vi "Write Subdiagram Labels.vi"(8 "Error In":errorcluster, 11 "DisableStructure In":refnum<vi>) -> (0 "Error Out":errorcluster, 3 "DisableStructure Out":refnum<vi>)   [LabVIEW 2017, in "Toolkit.lvlib"]
uses:
  Toolkit.lvlib
  Typedefs/Grave Frames.ctl
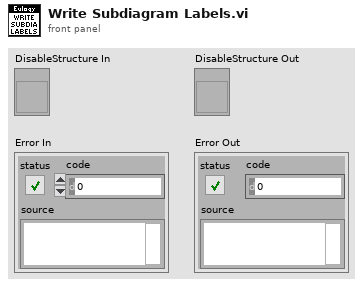
[diagram p1: front panel]
types:
  T1 = typedef "Toolkit.lvlib/Grave Frames.ctl" = enum16{"Corpse", "Spirit"}
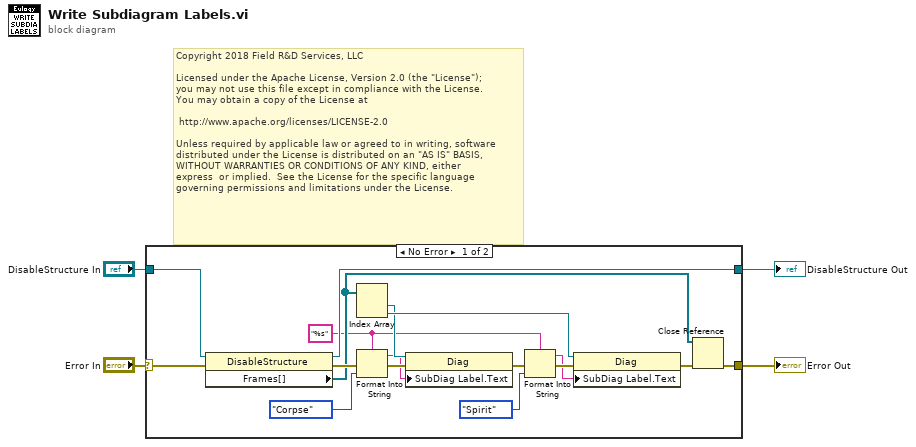
[diagram p0: block diagram]
diagram:
  # "Copyright 2018 Field R&D Services, LLC\n\nLicensed under the Apache License, Version 2.0 (the \"License\");\nyou may not use this file except in compliance with the License.\nYou may obtain a copy of the License at\n\n\thttp://www.apache.org/licenses/LICENSE-2.0\n\nUnless required by applicable law or agreed to in writing, software\ndistributed under the License is distributed on an \"AS IS\" BASIS,\nWITHOUT WARRANTIES OR CONDITIONS OF ANY KIND, either \nexpress  or implied.  See the License for the specific language \ngoverning permissions and limitations under the License."
  n1 = case shown="No Error" "Error In" {
    selector: "Error In" -> [w15 w22]
    tunnel: [w14 w22] -> w4
    tunnel: [w21 w23] -> w3
    tunnel: "DisableStructure In" -> [w17 w23]
    frame No Error {
      w7 = "%s" ("format string")
      n2 = property class="DisableStructure"(reference=w17, error in=w15) -> (reference out=w21:refnum<vi>, error out=w16:errorcluster, "Frames[]"=w12:refnum<vi>[])
      n3 = Index Array(array=w12) -> (element #1=w19:refnum<vi>, element #2=w20:refnum<vi>)  [unwired: 2 in]
      n4 = Format Into String(format string=w7, error in=w16, Grave_Frames."Corpse" ("Frame")) -> (resulting string=w9:string, error out=w11:errorcluster)  [unwired: 1 in]
      n5 = property class="Diag"(reference=w19, error in=w11, "SubDiag Label.Text"=w9) -> (error out=w18:errorcluster)  [unwired: 1 out]
      n6 = Format Into String(format string=w7, error in=w18, Grave_Frames."Spirit" ("Frame")) -> (resulting string=w5:string, error out=w8:errorcluster)  [unwired: 1 in]
      n7 = property class="Diag"(reference=w20, error in=w8, "SubDiag Label.Text"=w5) -> (error out=w13:errorcluster)  [unwired: 1 out]
      n8 = Close Reference(reference=w12, error in (no error)=w13) -> (error out=w14:errorcluster)
    }
    frame Error {
    }
  }
  "Error Out" <- w4
  "DisableStructure Out" <- w3
